vi "Open.vi"(8 "error in (no error)":errorcluster, 10 "Address":string, 11 "Example Instrument in":refnum<class "Instrument.Template.lvclass">) -> (0 "error out":errorcluster, 3 "Example Instrument out":refnum<class "Instrument.Template.lvclass">)   [LabVIEW 2019, in "Instrument.Template.lvclass"]
uses:
  Instrument.Template.lvclass
  Instrument Types/VSource/Instrument.VSource.lvclass
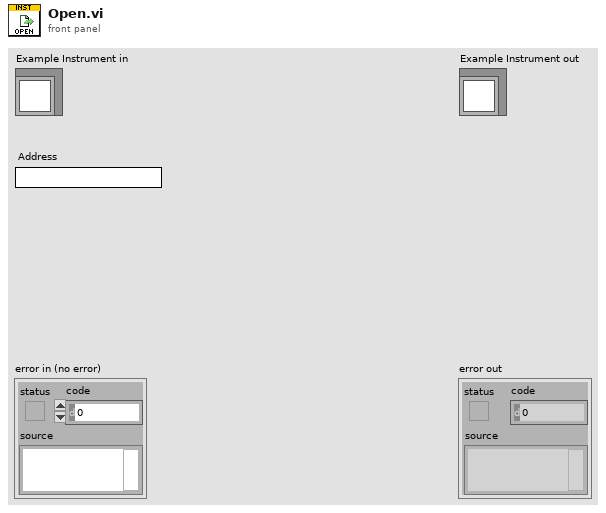
[diagram p1: front panel]
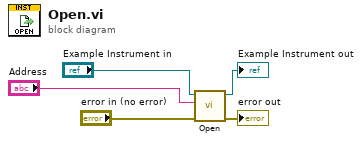
[diagram p0: block diagram]
diagram:
  n1 = call-parent "Open.vi"("error in (no error)"="error in (no error)", "Address"="Address", "Instrument in"="Example Instrument in") -> ("error out"=→"error out":errorcluster, "Instrument out"=→"Example Instrument out":refnum<class "Instrument.Template.lvclass">)  [unwired: 7 in]
